vi "Remove from Map.vi"(10 "key":refnum<class "IMessagePackObject.lvclass">, 11 "MsgPackMap in":refnum<class "MsgPackMap.lvclass">) -> (1 "value":refnum<class "IMessagePackObject.lvclass">, 2 "key not found?":bool, 3 "MsgPackMapout":refnum<class "MsgPackMap.lvclass">)   [LabVIEW 2020, in "MessagePack.lvlib" / "MsgPackMap.lvclass"]
uses:
  MsgPackMap.lvclass
  IMessagePackObject/IMessagePackObject.lvclass
  MsgPackMap.lvclass/MsgPackMap.ctl
  <vilib>/Utility/miscctls.llb/LVMapReplaceAction.ctl
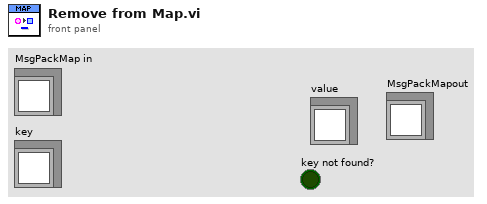
[diagram p1: front panel]
types:
  T1 = typedef "LVMapReplaceAction.ctl" = enum32{"Modify Entry only if found", "Add or Modify Entry", "Delete Entry"}
  T2 = map{refnum<class "IMessagePackObject.lvclass">, refnum<class "IMessagePackObject.lvclass">}
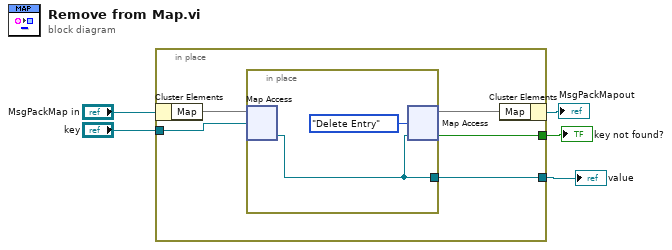
[diagram p0: block diagram]
diagram:
  n1 = in-place {
    in-place-border: "key" -> [w9]
    in-place-border: [w7] -> w3
    in-place-border: [w6] -> w1
    n2 = in-place-cluster #1("MsgPackMap in") -> ("Map"=w10:T2)
    n3 = in-place {
      in-place-border: [w11] -> w7
      n4 = in-place-map #2(w10, w9) -> (w11:refnum<class "IMessagePackObject.lvclass">)  [unwired: 1 in, 1 out]
      n5 = in-place-map #2(w11, LVMapReplaceAction."Delete Entry" ("action")) -> (w8:T2, w6:bool)  [unwired: 1 out]
    }
    n6 = in-place-cluster #1("Map"=w8) -> (→"MsgPackMapout":refnum<class "MsgPackMap.lvclass">)
  }
  "key not found?" <- w1
  "value" <- w3
